vi "runBECBasic.vi"() -> ()   [LabVIEW 2009, in "run.lvlib"]
doc: "Launch the applications that will control the experiment.\n\n1) Load Database, filesystem, file neologist.\n2) Start a clock for the DDS rf card.\n3) Launch Experiment Runner front viewer\n4) Launch Hardware Controller in the backend."
uses:
  run.lvlib
  Viewers/Editors/ExperimentRunner/ExperimentRunner.lvclass
  HWController/HWController.lvclass
  HWController/BECHWCBasic/BECHWCBasic.lvclass
  HWController/HWControllerEvents/HWControllerEvents.lvclass
  Tools/DatabaseHelpers/DbConnection/DeviceDataBase/deviceDataBase.lvclass
  HWController/HardwareConfiguration/HWConfiguration.lvclass
  Viewers/Editors/ExperimentRunner/RunExperiment/ExperimentControl.lvclass
  Viewers/Editors/ExperimentRunner/Events/ExperimentControlEvents.lvclass
  HWController/AtomChipHWC/AtomChipHWC.lvclass
  Tools/Filing/FileSystem/FileSystem.lvclass
  Tools/Filing/FileNeologist/FileNeologist.lvclass
  Tools/Filing.lvlib
  Tools/DatabaseHelpers.lvlib
  Events/Event.lvclass
  Viewers/ExperimentControl.lvlib
panel:
  in  "Experiment":enum16{"BEC1", "AtomChip"}(ring)=enum."AtomChip"
  in  "Camera on?":bool=TRUE
  in  "Hardware On?":bool=TRUE
  # "Hardware Off:\n\nWhen the HWController methods are called, make it change the status flag as normal, \nand simulate the changes of a real experiment to check the information flow."
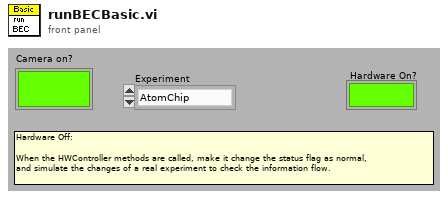
[diagram p1: front panel]
types:
  T1 = enum32{"Invalid", "Standard", "Closed", "Hidden", "Minimized", "Maximized"}
  T2 = enum32{"Bad", "Idle", "Run top level", "Running"}
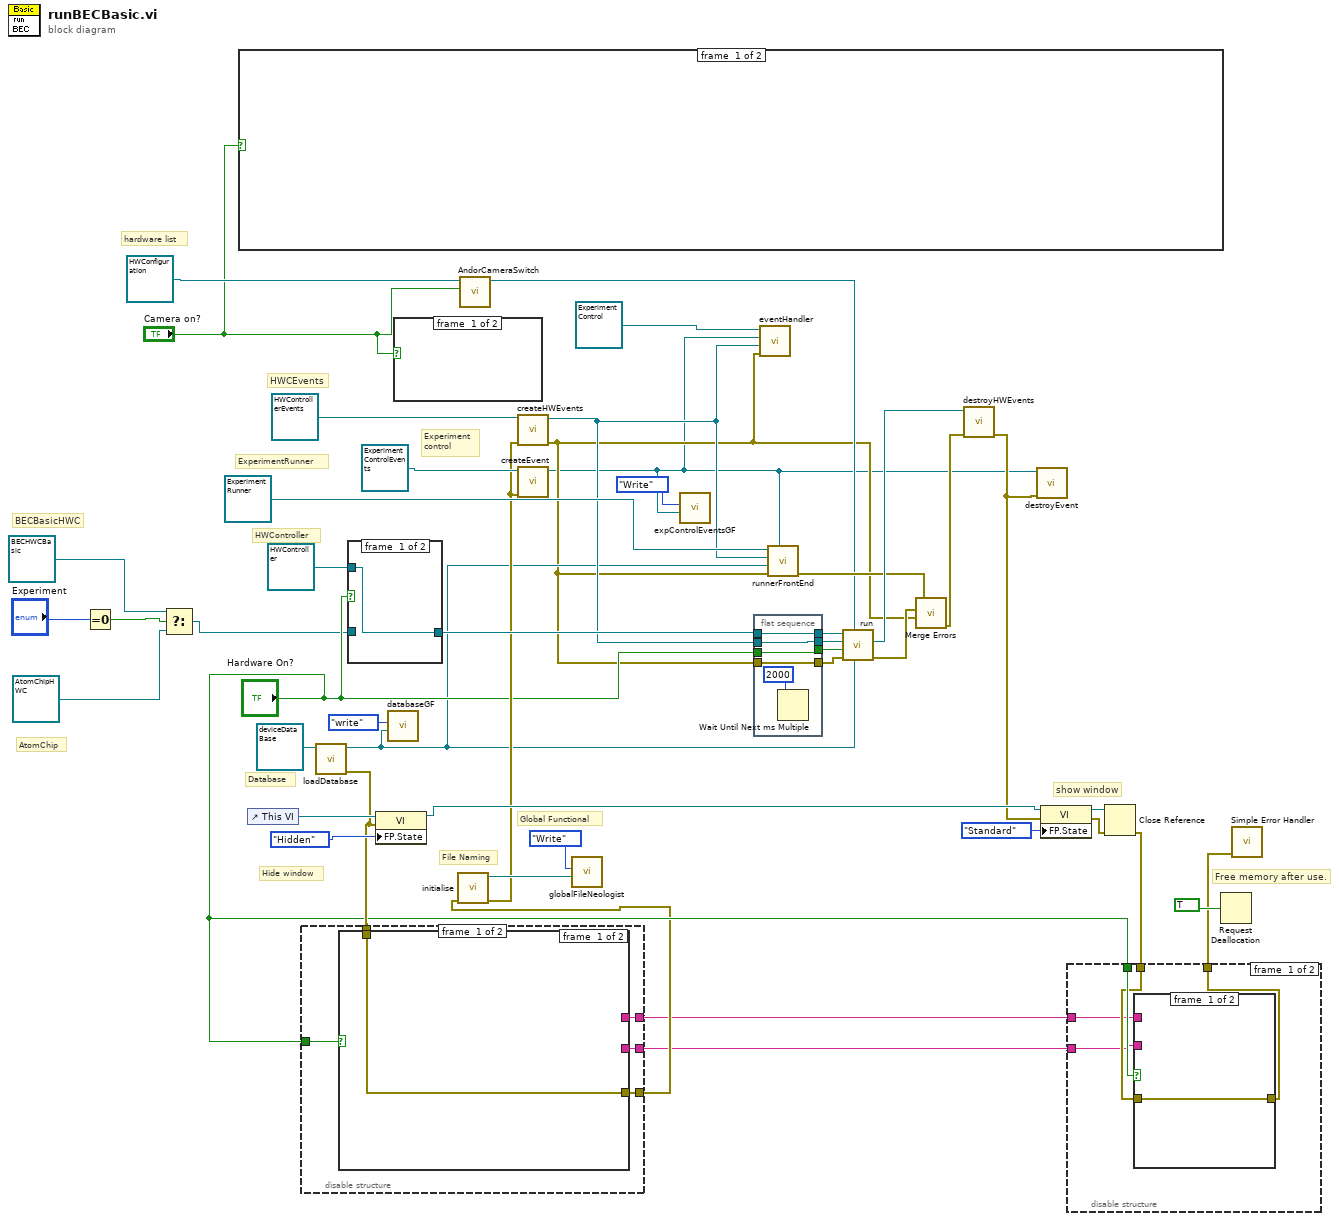
[diagram p0: block diagram]
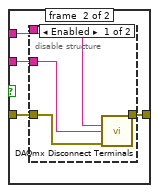
[diagram p2: hidden frame]
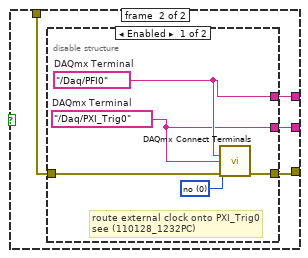
[diagram p5: hidden frame]
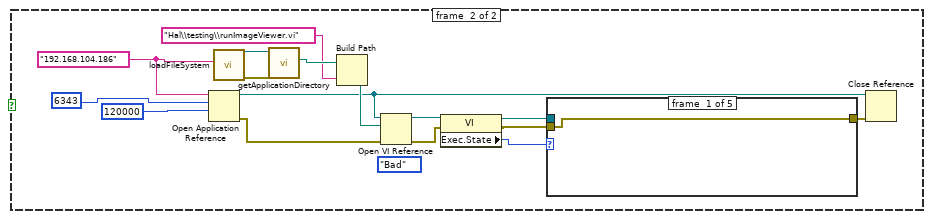
[diagram p8: hidden frame]
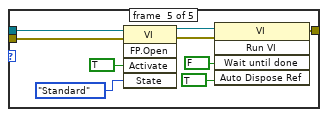
[diagram p12: hidden frame]
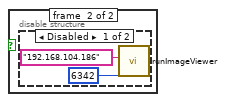
[diagram p13: hidden frame]
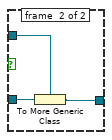
[diagram p15: hidden frame]
diagram:
  # "AtomChip"
  # "Experiment\ncontrol"
  # "hardware list"
  # "Free memory after use."
  # "BECBasicHWC"
  # "Hide window"
  # "show window"
  # "Database"
  # "File Naming"
  # "Global Functional"
  # "HWController"
  # "ExperimentRunner"
  # "HWCEvents"
  n1 = Equal To 0?(x="Experiment") -> (x = 0?=w7:bool)
  n2 = Select(t=refnum<class "BECHWCBasic.lvclass"> refnum ("Hardware:HWControllers.lvlib:BECHWCBasic.lvclass"), s=w7, f=refnum<class "AtomChipHWC.lvclass"> refnum ("Hardware:HWControllers.lvlib:AtomChipHWC.lvclass")) -> (s? t:f=w4:refnum<class "HWController.lvclass">)
  n3 = case shown="True" "Camera on?" {
    frame #0 {
    }
    frame #1 {
      (unwired) T2."Bad" ("Execution:State")
      w54 = "192.168.104.186" ("remote address")
      n4 = Open Application Reference(9:120000 ("timeout ms (60000)"), 10:6343, 11:w54) -> (0:w63:errorcluster, 3:w57:refnum<vi>)  [unwired: 1 in]
      n5 = call "loadFileSystem.vi"("computer name"=w54) -> ("error out"=w61:errorcluster, "FileSystem out"=w62:refnum<class "FileSystem.lvclass">)  [unwired: 9 in]
      n6 = call-dynamic "getApplicationDirectory.vi"("error in (no error)"=w61, "FileSystem.lvclass in"=w62) -> ("ApplicationDirectory"=w60:path)  [unwired: 7 in, 2 out]
      n7 = Build Path(base path=w60, name or relative path="Hal\\testing\\runImageViewer.vi") -> (appended path=w58:path)
      n8 = Open VI Reference(application reference (local)=w57, vi path=w58, error in (no error)=w63) -> (vi reference=w52:refnum<vi>, error out=w51:errorcluster)  [unwired: 3 in]
      n9 = property class="VI"(reference=w52, error in=w51) -> (reference out=w49:refnum<vi>, error out=w50:errorcluster, "Exec.State"=w48:T2)
      n10 = case shown="\"Idle\"" w48 {
        tunnel: [w64 w65 w66 w67 w74] -> w56
        tunnel: w50 -> [w64 w65 w66 w67 w69]
        tunnel: w49 -> [_ _ _ _ w68]
        frame #0 {
        }
        frame #1 {
        }
        frame #2 {
        }
        frame #3 {
        }
        frame #4 {
          n11 = invoke class="VI" method="FP.Open"(reference=w68, error in=w69, "Activate"=TRUE ("Activate?"), "State"=T1."Standard") -> (reference out=w70:refnum<vi>, error out=w71:errorcluster)  [unwired: 1 in, 3 out]
          n12 = invoke class="VI" method="Run VI"(reference=w70, error in=w71, "Wait until done"=FALSE, "Auto Dispose Ref"=TRUE ("Auto Dispose Reference")) -> (error out=w74:errorcluster)  [unwired: 1 in, 4 out]
        }
      }
      n13 = Close Reference(reference=w57, error in (no error)=w56) -> ()  [unwired: 1 out]
    }
  }
  n14 = control-ref of="This VI"() -> (w35:refnum<vi>)
  n15 = call "loadDatabase.vi"("deviceDataBase in"=refnum<class "deviceDataBase.lvclass"> refnum ("Tools.lvlib:DatabaseHelpers.lvlib:deviceDataBase.lvclass")) -> ("error out"=w18:errorcluster, "deviceDataBase out"=w10:refnum<class "deviceDataBase.lvclass">)  [unwired: 8 in, 1 out]
  n16 = disable-structure shown="Enabled" {
    disable-tunnel: w18 -> [w81 w93]
    disable-tunnel: "Hardware On?" -> [w80 _]
    disable-tunnel: [w79 w93] -> w16
    disable-tunnel: [w78 _] -> w13
    disable-tunnel: [w77 _] -> w12
    frame #0 {
      n17 = case shown="True" w80 {
        tunnel: w81 -> [w82 w86]
        tunnel: [w82 w85] -> w79
        tunnel: [_ w84] -> w78
        tunnel: [_ w83] -> w77
        frame #0 {
        }
        frame #1 {
          n18 = disable-structure shown="Enabled" {
            disable-tunnel: w86 -> [w90 w92]
            disable-tunnel: [w89 w92] -> w85
            disable-tunnel: [w88 _] -> w84
            disable-tunnel: [w87 _] -> w83
            frame #0 {
              w91 = 0 items=["no", "yes"] ("invert polarity")
              w87 = tag "/Daq/PXI_Trig0"  # DAQmx Terminal
              w88 = tag "/Daq/PFI0"  # DAQmx Terminal
              # "route external clock onto PXI_Trig0\nsee (110128_1232PC)"
              n19 = call <vilib>:"DAQmx Connect Terminals.vi"("source terminal"=w88, "destination terminal"=w87, "invert polarity"=w91, "error in"=w90) -> ("error out"=w89:errorcluster)  [unwired: 11 in]
            }
            frame #1 {
            }
          }
        }
      }
    }
    frame #1 {
    }
  }
  n20 = case shown="True" "Hardware On?" {
    tunnel: w4 -> [_ w97]
    tunnel: refnum<class "HWController.lvclass"> refnum ("Hardware:HWControllers.lvlib:HWController.lvclass") -> [w94 w96]
    tunnel: [w94 w95] -> w38
    frame #0 {
    }
    frame #1 {
      n21 = To More Generic Class(target class=w96, reference=w97) -> (generic class reference=w95:refnum<class "HWController.lvclass">)
    }
  }
  n22 = property class="VI"(reference=w35, error in=w18, "FP.State"=T1."Hidden" ("Front Panel Window:State")) -> (reference out=w26:refnum<vi>)  [unwired: 1 out]
  n23 = call "databaseGF.vi"("deviceDataBase in"=w10, "Enum"=enum16{"write", "read"}."write") -> ()  [unwired: 9 in, 1 out]
  n24 = case shown="True" "Camera on?" {
    frame #0 {
    }
    frame #1 {
      n25 = disable-structure shown="Disabled" {
        frame #0 {
          n26 = call "runImageViewer.vi"("remote port"=u16 6342, "remote address"="192.168.104.186") -> ()  [unwired: 10 in]
        }
        frame #1 {
        }
      }
    }
  }
  n27 = call "initialise.vi"("error in (no error)"=w16) -> ("error out"=w21:errorcluster, "FileNeologist out"=w30:refnum<class "FileNeologist.lvclass">)  [unwired: 9 in]
  n28 = call "AndorCameraSwitch.vi"("Andor Camera"="Camera on?", "HWConfiguration in"=refnum<class "HWConfiguration.lvclass"> refnum ("HardwareList out")) -> ("HWConfiguration out"=w23:refnum<class "HWConfiguration.lvclass">)  [unwired: 8 in, 1 out]
  n29 = call-dynamic "createHWEvents.vi"("error in (no error)"=w21, "HWControllerEvents in"=refnum<class "HWControllerEvents.lvclass"> refnum ("Hardware:HWControllers.lvlib:HWControllerEvents.lvclass")) -> ("error out"=w9:errorcluster, "HWControllerEvents out"=w11:refnum<class "HWControllerEvents.lvclass">)  [unwired: 8 in]
  n30 = call "createEvent.vi"("error in (no error)"=w21, "Event in"=refnum<class "ExperimentControlEvents.lvclass"> refnum ("ExperimentControlEvents")) -> ("Event out"=w2:refnum<class "ExperimentControlEvents.lvclass">)  [unwired: 8 in, 1 out]
  n31 = call "globalFileNeologist.vi"("FileNeologist in"=w30, "Action"=enum16{"Write", "Read"}."Write") -> ()  [unwired: 9 in, 1 out]
  n32 = call "expControlEventsGF.vi"("ExperimentControlEvents"=w2, "Action"=enum16{"Write", "Read"}."Write") -> ()  [unwired: 9 in, 1 out]
  n33 = flat-sequence {
    tunnel: [w103] -> w40
    tunnel: [w104] -> w39
    tunnel: w38 -> [w104]
    tunnel: w11 -> [w103]
    tunnel: [w102] -> w37
    tunnel: "Hardware On?" -> [w102]
    tunnel: [w101] -> w36
    tunnel: w9 -> [w101]
    frame #0 {
      n34 = Wait Until Next ms Multiple(millisecond multiple=2000) -> ()  [unwired: 1 out]
    }
  }
  n35 = call "eventHandler.vi"("error in (no error)"=w9, ":HWControllerEvents"=w11, "ExperimentControlEvents"=w2, "ExperimentControl in"=refnum<class "ExperimentControl.lvclass"> refnum) -> ()  [unwired: 6 in, 2 out]
  n36 = call "runnerFrontEnd.vi"("ExperimentControlEvents"=w2, "error in (no error)"=w9, "deviceDataBase"=w10, "HWControllerEvents"=w11, "Views.lvlib:ExperimentControl.lvlib:ExperimentRunner in"=refnum<class "ExperimentRunner.lvclass"> refnum ("Views.lvlib:ExperimentControl.lvlib:ExperimentRunner.lvclass")) -> ("error out"=w44:errorcluster)  [unwired: 5 in, 1 out]
  n37 = call "run.vi"("deviceDatabase"=w10, "HardwareList out"=w23, "error in (no error)"=w36, "debuggingFlag"=w37, "HWControllerEvents"=w40, "HWController in"=w39) -> ("error out"=w43:errorcluster, "HWControllerEvents out"=w45:refnum<class "HWControllerEvents.lvclass">)  [unwired: 3 in, 1 out]
  n38 = call <vilib>:"Merge Errors.vi"("error in 3 (no error)"=w9, "error in 2 (no error)"=w43, "error in 1 (no error)"=w44) -> ("error out"=w42:errorcluster)  [unwired: 4 in]
  n39 = call-dynamic "destroyHWEvents.vi"("error in (no error)"=w42, "HWControllerEvents in"=w45) -> ("error out"=w20:errorcluster)  [unwired: 8 in, 1 out]
  n40 = call "destroyEvent.vi"("error in (no error)"=w20, "Event in"=w2) -> ()  [unwired: 8 in, 2 out]
  n41 = property class="VI"(reference=w26, error in=w20, "FP.State"=T1."Standard" ("Front Panel Window:State")) -> (reference out=w31:refnum<vi>, error out=w32:errorcluster)
  n42 = Close Reference(reference=w31, error in (no error)=w32) -> (error out=w15:errorcluster)
  n43 = disable-structure shown="Enabled" {
    disable-tunnel: "Hardware On?" -> [w109 _]
    disable-tunnel: w15 -> [w108 w120]
    disable-tunnel: [w107 w120] -> w14
    disable-tunnel: w13 -> [w106 _]
    disable-tunnel: w12 -> [w105 _]
    frame #0 {
      n44 = case shown="True" w109 {
        tunnel: w108 -> [w110 w114]
        tunnel: [w110 w113] -> w107
        tunnel: w106 -> [_ w112]
        tunnel: w105 -> [_ w111]
        frame #0 {
        }
        frame #1 {
          n45 = disable-structure shown="Enabled" {
            disable-tunnel: w114 -> [w118 w119]
            disable-tunnel: [w117 w119] -> w113
            disable-tunnel: w112 -> [w116 _]
            disable-tunnel: w111 -> [w115 _]
            frame #0 {
              n46 = call <vilib>:"DAQmx Disconnect Terminals.vi"("source terminal"=w116, "destination terminal"=w115, "error in"=w118) -> ("error out"=w117:errorcluster)  [unwired: 12 in]
            }
            frame #1 {
            }
          }
        }
      }
    }
    frame #1 {
    }
  }
  n47 = Request Deallocation(TRUE) -> ()
  n48 = call <vilib>:"Simple Error Handler.vi"("error in (no error)"=w14) -> ()  [unwired: 4 in, 5 out]
